vi "tagDB_Value_Template_RegExp_Ref.vi"(8 "error in (no error)":errorcluster, 9 "Type":refnum<vi>, 10 "RegExp":string, 11 "DB Ref":T1) -> (0 "error out":errorcluster, 1 "names":string[](array[string]), 2 "value":refnum<vi>[](array[refnum]), 3 "DB Ref(dup)":T1)   [LabVIEW 2014, in "TagDB(dev).lvlib"]
doc: "[Covers: REQ_TAGDB_TEMPLATE_VALUE_REGEXP_REF]"
uses:
  tagDB_Def.ctl
  Error/_[error50001]Can't Found Value.vi
  Private/_Cast TagDB Ref to DVR.vi
  _global/URL/TRIM-BOTH-SPACE.vi
  Error/_[error50000]Invalid DB REF.vi
  TagDB(dev).lvlib
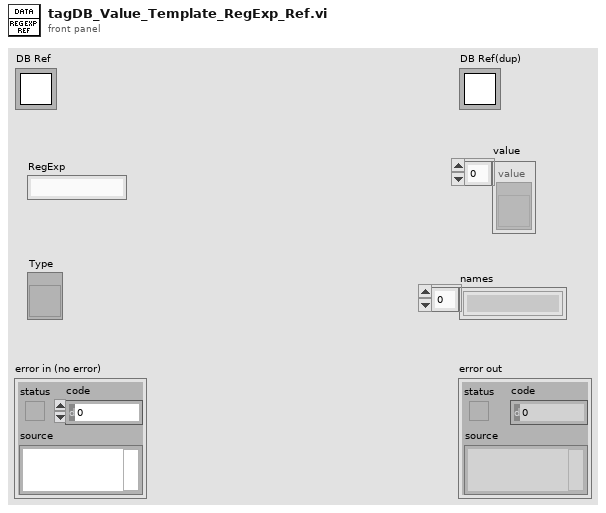
[diagram p1: front panel]
types:
  T1 = typedef "TagDB(dev).lvlib/tagDB_Def.ctl" = refnum<k1>
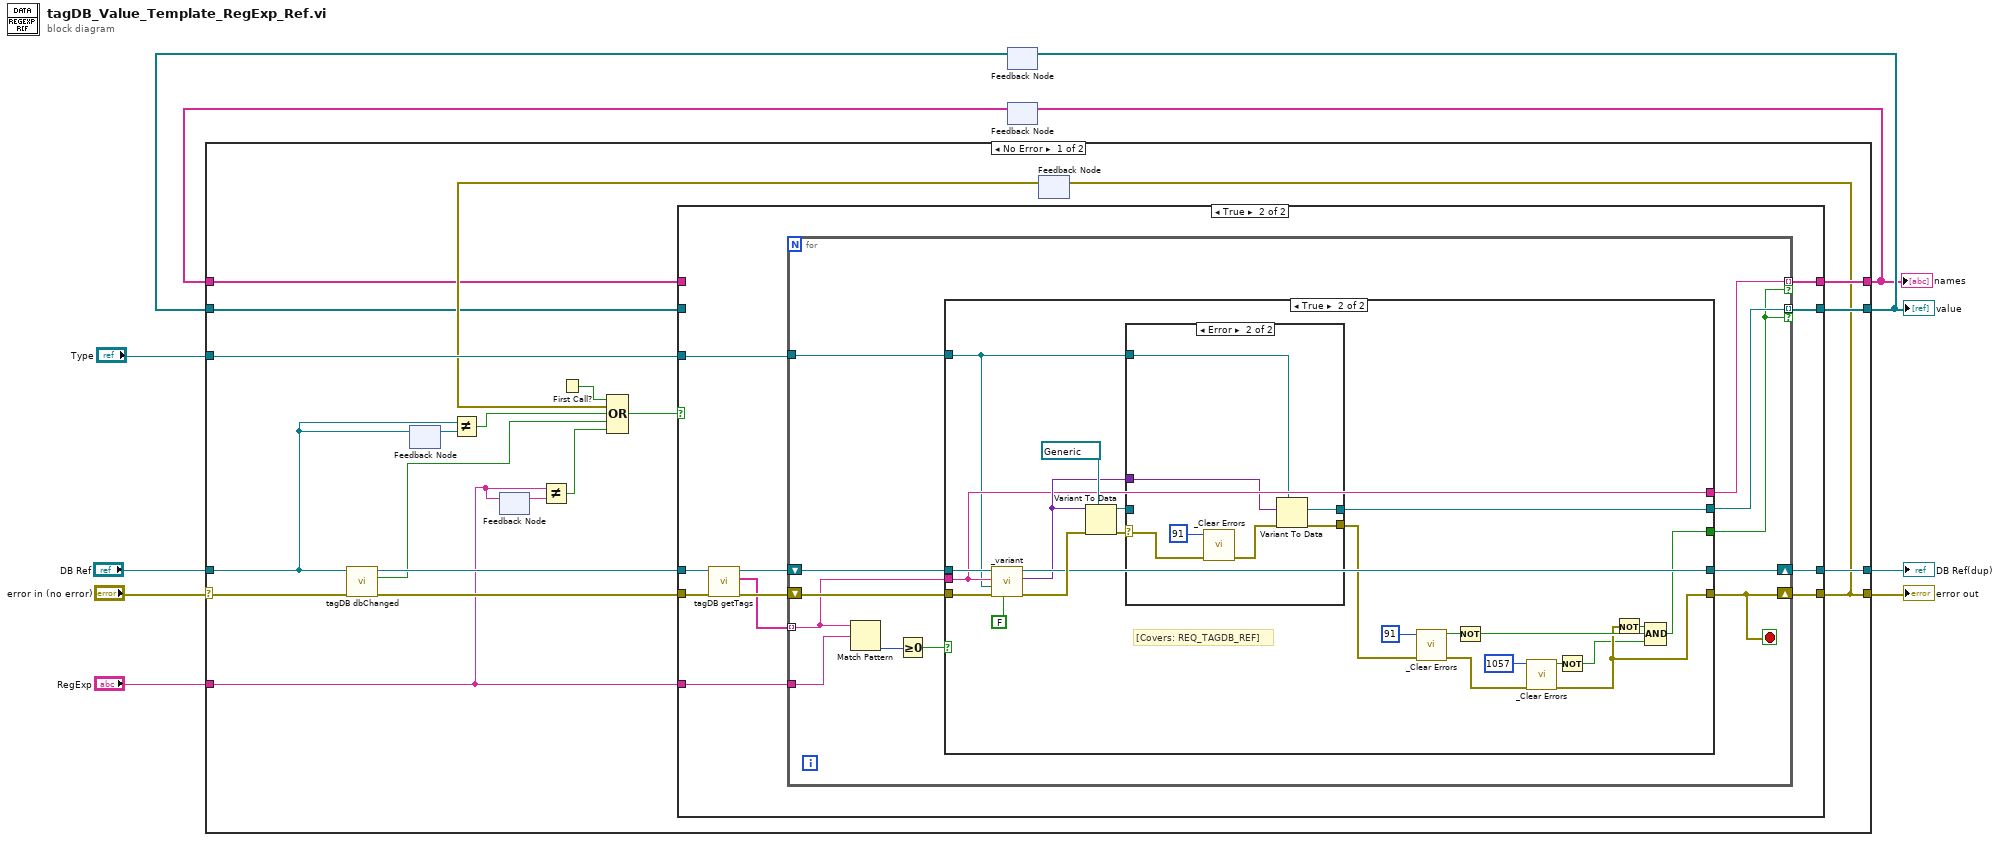
[diagram p0: block diagram]
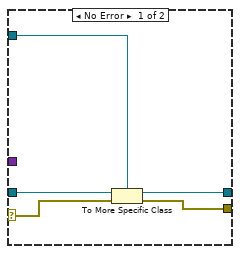
[diagram p4: hidden frame]
diagram:
  n1 = feedback #1() -> (w2:refnum<vi>[])  [unwired: 1 in]
  n2 = feedback #2() -> (w3:string[])  [unwired: 1 in]
  n3 = case shown="No Error" "error in (no error)" {
    selector: "error in (no error)" -> [w25 w99]
    tunnel: [w15 w99] -> w9
    tunnel: [w30 w98] -> w7
    tunnel: "DB Ref" -> [w16 w98]
    tunnel: "RegExp" -> [w17 _]
    tunnel: "Type" -> [w28 _]
    tunnel: [w29 w96] -> w5
    tunnel: [w27 w97] -> w4
    tunnel: w3 -> [w12 w97]
    tunnel: w2 -> [w11 w96]
    frame No Error {
      n4 = call "tagDB dbChanged.vi"("error in (no error)"=w25, "DB Ref"=w16) -> ("error in (no error) (dup)"=w24:errorcluster, "changed?"=w18:bool, "DB Ref (dup)"=w26:T1)  [unwired: 7 in]
      n5 = feedback #3() -> (w22:T1)  [unwired: 1 in]
      n6 = feedback-in #3(w16) -> ()
      n7 = Not Equal?(x=w16, y=w22) -> (x != y?=w20:bool)
      n8 = feedback #4() -> (w21:string)  [unwired: 1 in]
      n9 = feedback-in #4(w17) -> ()
      n10 = Not Equal?(x=w17, y=w21) -> (x != y?=w19:bool)
      n11 = First Call?() -> (First Call?: T/F=w23:bool)
      n12 = feedback #5() -> (w14:errorcluster)  [unwired: 1 in]
      n13 = Compound Arithmetic op=OR(w23, w14, w20, w18, w19) -> (w13:bool)
      n14 = case shown="True" w13 {
        tunnel: [w32 w45] -> w30
        tunnel: [w33 w44] -> w29
        tunnel: w28 -> [_ w43]
        tunnel: [w34 w39] -> w27
        tunnel: w26 -> [w32 w38]
        tunnel: w24 -> [w31 w37]
        tunnel: w17 -> [_ w36]
        tunnel: [w31 w35] -> w15
        tunnel: w12 -> [w34 _]
        tunnel: w11 -> [w33 _]
        frame False {
        }
        frame True {
          n15 = call "tagDB getTags.vi"("error in (no error)"=w37, "DB Ref in"=w38) -> ("error out"=w41:errorcluster, "DB items"=w40:string[], "DB Ref out"=w42:T1)  [unwired: 7 in]
          n16 = for {
            tunnel: w36 -> [w52]
            shift-right: [w57] -> w45
            shift-left: w42 -> [w55]
            shift-right: [w50] -> w35
            shift-left: w41 -> [w54]
            tunnel: w43 -> [w53]
            tunnel: [w56] -> w44 mode=indexing if=w48
            tunnel: w40 -> [w47] mode=indexing
            tunnel: [w49] -> w39 mode=indexing if=w48
            stop <- w50 stop-if-true
            n17 = Match Pattern(string=w47, regular expression=w52) -> (offset past match=w46:i32)  [unwired: 1 in, 3 out]
            n18 = Greater Or Equal To 0?(x=w46) -> (x >= 0?=w51:bool)
            n19 = case shown="True" w51 {
              tunnel: [w59 w66] -> w50
              tunnel: [w60 w82] -> w57
              tunnel: [w58 w73] -> w56
              tunnel: w55 -> [w60 w81]
              tunnel: w54 -> [w59 w80]
              tunnel: w53 -> [w58 w62]
              tunnel: [_ w76] -> w48
              tunnel: [_ w64] -> w49
              tunnel: w47 -> [_ w64]
              frame False {
              }
              frame True {
                # "[Covers: REQ_TAGDB_REF]"
                n20 = call "_variant.vi"("Add wih NonExist?"=FALSE, "error in (no error)"=w80, "default value (empty variant)"=w62, "name"=w64, "DB Ref"=w81) -> ("error out"=w83:errorcluster, "value"=w70:variant, "DB Ref (dup)"=w82:T1)  [unwired: 4 in]
                n21 = Variant To Data(error in=w83, type=refnum<vi> refnum ("value"), Variant=w70) -> (data=w72:refnum<vi>, error out=w63:errorcluster)
                n22 = case shown="Error" w63 {
                  selector: w63 -> [w86 w95]
                  tunnel: [w87 w90] -> w73
                  tunnel: [w85 w92] -> w71
                  tunnel: w62 -> [w84 w91]
                  tunnel: w72 -> [w88 _]
                  tunnel: w70 -> [_ w89]
                  frame No Error {
                    n23 = To More Specific Class(target class=w84, reference=w88, error in=w86) -> (specific class reference=w87:refnum<vi>, error out=w85:errorcluster)
                  }
                  frame Error {
                    n24 = call "_Clear Errors.vi"("error in (no error)"=w95, "specific error code to clear (0: all)"=91) -> ("error out"=w93:errorcluster)  [unwired: 4 in, 1 out]
                    n25 = Variant To Data(error in=w93, type=w91, Variant=w89) -> (data=w90:refnum<vi>, error out=w92:errorcluster)
                  }
                }
                n26 = call "_Clear Errors.vi"("error in (no error)"=w71, "specific error code to clear (0: all)"=91) -> ("error out"=w67:errorcluster, "specific error cleared?"=w78:bool)  [unwired: 4 in]
                n27 = Not(x=w78) -> (.not. x?=w77:bool)
                n28 = call "_Clear Errors.vi"("error in (no error)"=w67, "specific error code to clear (0: all)"=1057) -> ("error out"=w66:errorcluster, "specific error cleared?"=w69:bool)  [unwired: 4 in]
                n29 = Not(x=w69) -> (.not. x?=w65:bool)
                n30 = Not(x=w66) -> (.not. x?=w75:bool)
                n31 = Compound Arithmetic op=AND(w75, w77, w65) -> (w76:bool)
              }
            }
          }
        }
      }
      n32 = feedback-in #5(w15) -> ()
    }
    frame Error {
    }
  }
  "error out" <- w9
  "DB Ref(dup)" <- w7
  "value" <- w5
  "names" <- w4
  n33 = feedback-in #1(w5) -> ()
  n34 = feedback-in #2(w4) -> ()
